vi "Check Register Data Store.vi"(8 "error in (no error)":errorcluster, 10 "register name":string, 11 "register data store in":T1) -> (0 "error IO":errorcluster, 1 "Found":bool, 2 "register offset":u32, 3 "register data store out":T1)   [LabVIEW 2026, in "FPGA Register IO.lvlib"]
uses:
  FPGA Register IO.lvlib
  TypeDefs/Register Data Store.ctl
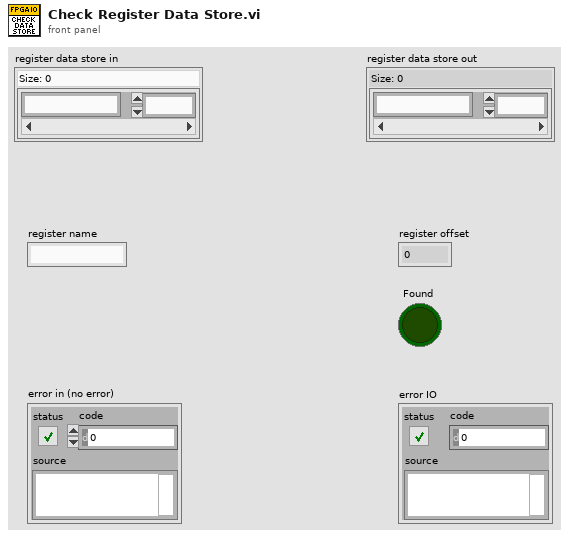
[diagram p1: front panel]
types:
  T1 = typedef "FPGA Register IO.lvlib/Register Data Store.ctl" = map{string, u32}
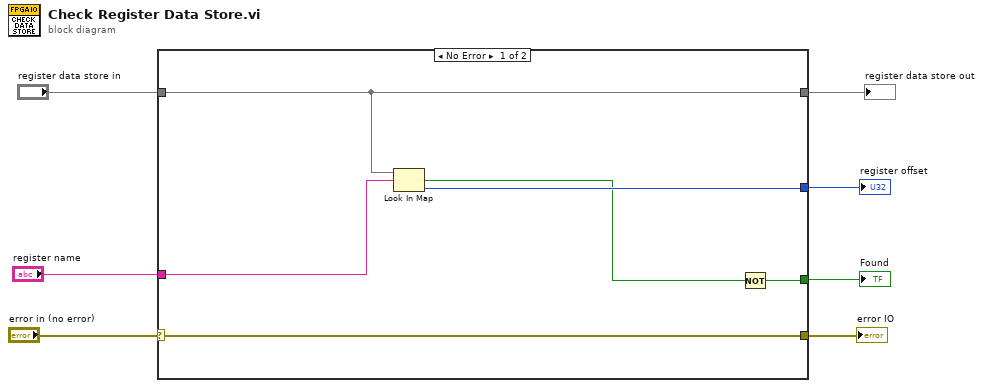
[diagram p0: block diagram]
diagram:
  n1 = case shown="No Error" "error in (no error)" {
    selector: "error in (no error)" -> [w13 w15]
    tunnel: "register name" -> [w11 _]
    tunnel: "register data store in" -> [w12 w14]
    tunnel: [w10 _] -> w1
    tunnel: [w8 _] -> w5
    tunnel: [w12 w14] -> w3
    tunnel: [w13 w15] -> w2
    frame No Error {
      n2 = Look In Map(map=w12, key=w11) -> (key not found?=w9:bool, value=w10:u32)  [unwired: 1 in]
      n3 = Not(x=w9) -> (.not. x?=w8:bool)
    }
    frame Error {
    }
  }
  "register offset" <- w1
  "register data store out" <- w3
  "Found" <- w5
  "error IO" <- w2
